vi "staticcoord.vi"() -> ()   [LabVIEW 2012]
uses:
  <vilib>/vision/NI_Vision_Development_Module.lvlib
panel:
  in  "Settings":T1={"Objects"=0, "Threshold"=128, "Reject Border"=FALSE, "Fill Holes"=FALSE, "Min Object Size"=FALSE, "Min Size"=3, "Max Object Size"=FALSE, "Max Size"=100, "Show Search Area"=FALSE, "Show Center"=TRUE, "Show Bounding Box"=TRUE} {"Objects" items=["Bright Objects", "Dark Objects"]; "Threshold" min=1 max=999999999 step=1; "Max Size" min=1 max=999999999 step=1; "Min Size" min=1 max=999999999 step=1}
  out "String":string
  out "Image Out 2":T2(plugin-control)
  out "Image Out":T2(plugin-control)
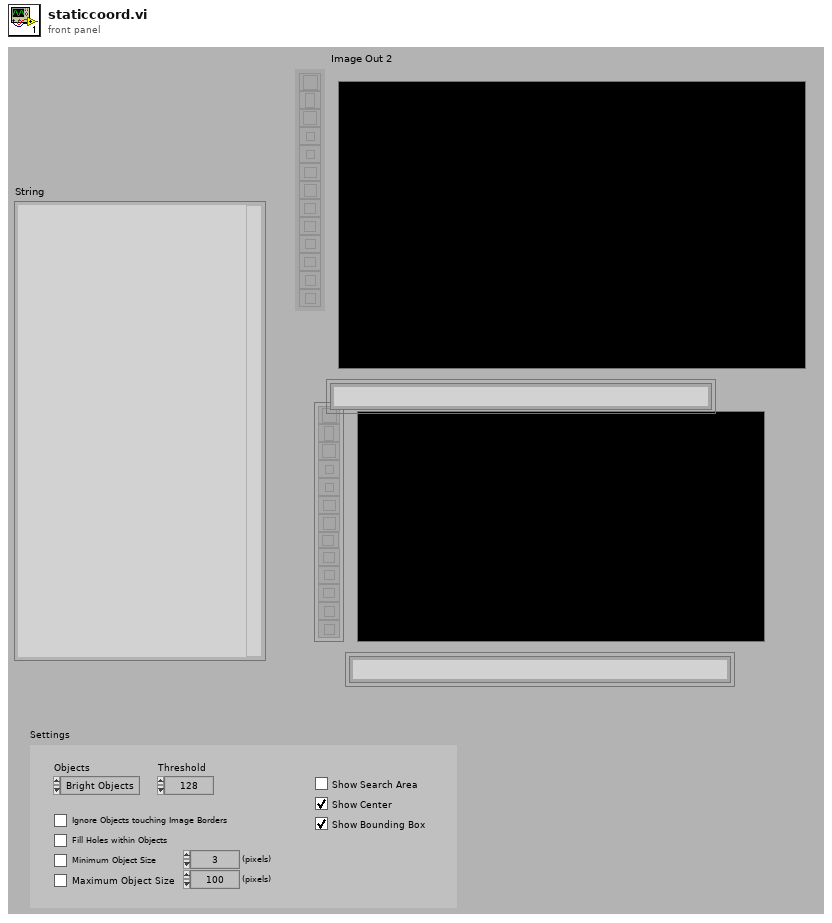
[diagram p1: front panel]
types:
  T1 = cluster{"Objects":u16, "Threshold":i32, "Reject Border":bool, "Fill Holes":bool, "Min Object Size":bool, "Min Size":i32, "Max Object Size":bool, "Max Size":i32, "Show Search Area":bool, "Show Center":bool, "Show Bounding Box":bool}
  T2 = typedef "IMAQ Image.ctl" = refnum<image>
  T3 = cluster{"Object Center":cluster{"X":sgl, "Y":sgl}, "Bounding Box":cluster{"X Left":i32, "Y Top":i32, "X Right":i32, "Y Bottom":i32}, "Area":sgl, "Orientation":sgl, "Aspect Ratio":sgl, "Nb Holes":i32}[]
  T4 = cluster{"Object Center":cluster{"X":sgl, "Y":sgl}, "Bounding Box":cluster{"X Left":i32, "Y Top":i32, "X Right":i32, "Y Bottom":i32}, "Area":sgl, "Orientation":sgl, "Aspect Ratio":sgl, "Nb Holes":i32}
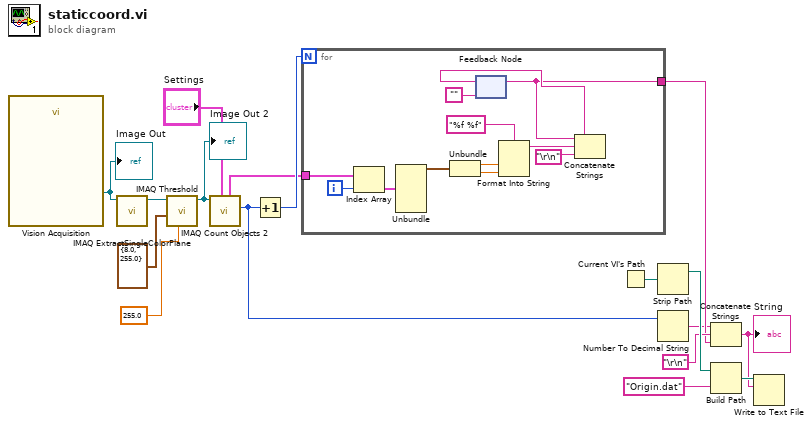
[diagram p0: block diagram]
diagram:
  n1 = call "Vision Acquisition"() -> ("Image Out"=w2:T2)  [unwired: 26 in, 1 out]
  "Image Out" <- w2
  n2 = call "IMAQ ExtractSingleColorPlane"("Image Src"=w2) -> ("Image Dst Out"=w15:T2)  [unwired: 9 in, 1 out]
  n3 = call "IMAQ Threshold"("Replace Value"=sgl 255.0 ("replace value"), "Range"=cluster{"lower value":sgl, "upper value":sgl} {"lower value"=8.0, "upper value"=255.0} ("threshold"), "Image Src"=w15) -> ("Image Dst Out"=w4:T2)  [unwired: 7 in, 1 out]
  "Image Out 2" <- w4
  n4 = call "IMAQ Count Objects 2"("Settings"="Settings", "Image"=w4) -> ("Number of Objects"=w3:i32, "Objects"=w5:T3)  [unwired: 5 in, 3 out]
  n5 = Increment(x=w3) -> (x+1=w9:i32)
  n6 = for {
    N: w9 -> [_]
    tunnel: w5 -> [w29]
    tunnel: [w21] -> w8
    i -> [w24]
    n7 = Index Array(array=w29, index=w24) -> (element=w28:T4)
    n8 = Unbundle(w28) -> ("Object Center"=w27:cluster{"X":sgl, "Y":sgl})  [unwired: 5 out]
    n9 = Unbundle(w27) -> ("X"=w18:sgl, "Y"=w19:sgl)
    n10 = feedback #1("") -> (w21:string)
    n11 = Format Into String(format string="%f %f", w18, w19) -> (resulting string=w23:string)  [unwired: 2 in, 1 out]
    n12 = Concatenate Strings(w21, w23, "\r\n") -> (w22:string)
    n13 = feedback-in #1(w22) -> ()
  }
  n14 = Current VI's Path() -> (path=w13:path)
  n15 = Strip Path(path=w13) -> (stripped path=w11:path)  [unwired: 1 out]
  n16 = Number To Decimal String(number=w3) -> (decimal integer string=w7:string)  [unwired: 1 in]
  n17 = Concatenate Strings(w7, "\r\n", w8) -> (w6:string)
  "String" <- w6
  n18 = Build Path(base path=w11, name or relative path="Origin.dat" ("standard input")) -> (appended path=w14:path)
  n19 = Write to Text File(file (use dialog)=w14, text=w6) -> ()  [unwired: 2 in, 3 out]
